vi "OverSample.vi"(2 "delay":sgl, 3 "raw data in":dbl[][](array[numeric]) format="%.2f", 4 "Add Lines":u16=1, 5 "reduce RF pts by factor of":i32=4) -> (1 "reduced data out":dbl[][](array[numeric]) format="%.2f")   [LabVIEW 2022 SP3]
uses:
  <vilib>/Analysis/2dsp.llb/Decimate (single shot, DBL).vi
  <vilib>/Analysis/NI_AALPro.lvlib
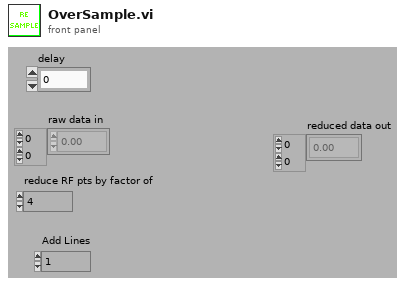
[diagram p1: front panel]
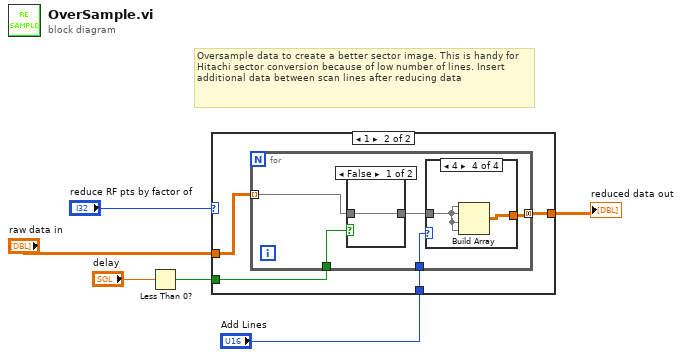
[diagram p0: block diagram]
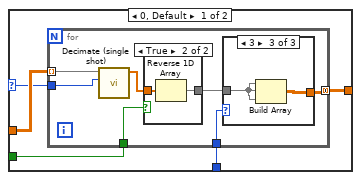
[diagram p2: hidden frame]
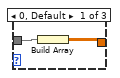
[diagram p3: hidden frame]
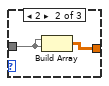
[diagram p4: hidden frame]
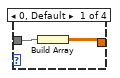
[diagram p6: hidden frame]
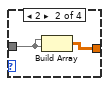
[diagram p7: hidden frame]
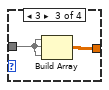
[diagram p8: hidden frame]
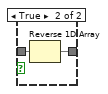
[diagram p9: hidden frame]
diagram:
  # "Oversample data to create a better sector image. This is handy for Hitachi sector conversion because of low number of lines. Insert additional data between scan lines after reducing data"
  n1 = Less Than 0?(x="delay") -> (x < 0?=w6:bool)
  n2 = case shown="1" "reduce RF pts by factor of" {
    selector: "reduce RF pts by factor of" -> [w9 _]
    tunnel: [w10 w30] -> w2
    tunnel: "raw data in" -> [w11 w31]
    tunnel: w6 -> [w8 w29]
    tunnel: "Add Lines" -> [w7 w28]
    frame 0, Default {
      n3 = for {
        tunnel: w11 -> [w18] mode=indexing
        tunnel: [w12] -> w10 mode=concatenating
        tunnel: w9 -> [w17]
        tunnel: w8 -> [w16]
        tunnel: w7 -> [w14]
        n4 = call-poly <vilib>:"Decimate (single shot).vi"("decimating factor"=w17, "X"=w18) -> ("Decimated Array"=w15:dbl[])  [unwired: 8 in, 1 out]
        n5 = case shown="True" w16 {
          tunnel: w15 -> [w25 w27]
          tunnel: [w25 w26] -> w13
          frame False {
          }
          frame True {
            n6 = Reverse 1D Array(array=w27) -> (reversed array=w26:dbl[])
          }
        }
        n7 = case shown="3" w14 {
          tunnel: [w19 w21 w24] -> w12
          tunnel: w13 -> [w20 w22 w23]
          frame 0, Default {
            n8 = Build Array(w20) -> (w19:dbl[][])
          }
          frame 2 {
            n9 = Build Array(w22, w22) -> (w21:dbl[][])
          }
          frame 3 {
            n10 = Build Array(w23, w23, w23) -> (w24:dbl[][])
          }
        }
      }
    }
    frame 1 {
      n11 = for {
        tunnel: w31 -> [w32] mode=indexing
        tunnel: [w33] -> w30 mode=concatenating
        tunnel: w29 -> [w36]
        tunnel: w28 -> [w35]
        n12 = case shown="False" w36 {
          tunnel: w32 -> [w45 w47]
          tunnel: [w45 w46] -> w34
          frame False {
          }
          frame True {
            n13 = Reverse 1D Array(array=w47) -> (reversed array=w46:dbl[])
          }
        }
        n14 = case shown="4" w35 {
          tunnel: [w37 w39 w42 w44] -> w33
          tunnel: w34 -> [w38 w40 w41 w43]
          frame 0, Default {
            n15 = Build Array(w38) -> (w37:dbl[][])
          }
          frame 2 {
            n16 = Build Array(w40, w40) -> (w39:dbl[][])
          }
          frame 3 {
            n17 = Build Array(w41, w41, w41) -> (w42:dbl[][])
          }
          frame 4 {
            n18 = Build Array(w43, w43, w43, w43) -> (w44:dbl[][])
          }
        }
      }
    }
  }
  "reduced data out" <- w2
